vi "set_pixel_dwell_time.vi"(8 "error in (no error)":errorcluster, 10 "Pixel dwell time":dbl=719.0, 11 "TrajectoryRK110428Fiber in":refnum<class "TrajectoryRK110428Fiber_Spiral.lvclass">) -> (0 "error out":errorcluster, 3 "TrajectoryRK110428Fiber out":refnum<class "TrajectoryRK110428Fiber_Spiral.lvclass">)   [LabVIEW 2010, in "TrajectoryRK110428Fiber_Spiral.lvclass"]
uses:
  TrajectoryRK110428Fiber_Spiral.lvclass
  TrajectoryRK110428Fiber_Spiral.lvclass/TrajectoryRK110428Fiber_Spiral.ctl
panel:
  # "[µs]"
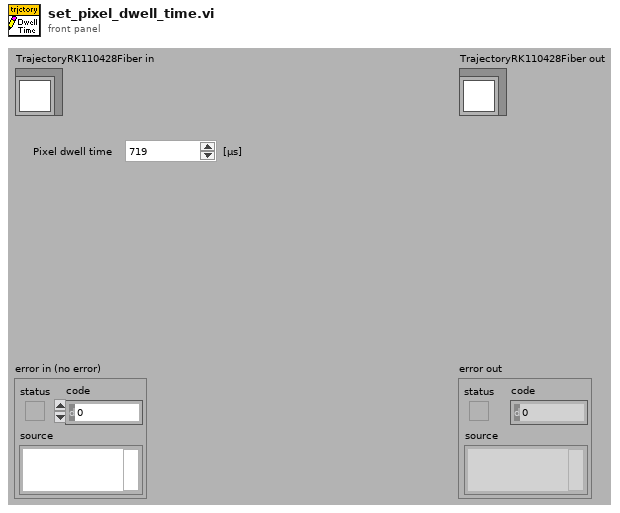
[diagram p1: front panel]
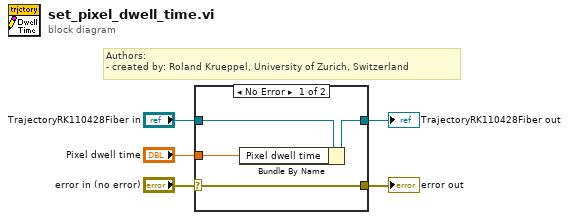
[diagram p0: block diagram]
diagram:
  # "Authors: \n- created by: Roland Krueppel, University of Zurich, Switzerland"
  n1 = case shown="No Error" "error in (no error)" {
    selector: "error in (no error)" -> [w9 w10]
    tunnel: [w9 w10] -> w4
    tunnel: [w7 w11] -> w2
    tunnel: "TrajectoryRK110428Fiber in" -> [w8 w11]
    tunnel: "Pixel dwell time" -> [w6 _]
    frame No Error {
      n2 = Bundle By Name(cluster=w8, "Pixel dwell time"=w6) -> (w7:refnum<class "TrajectoryRK110428Fiber_Spiral.lvclass">)
    }
    frame Error {
    }
  }
  "error out" <- w4
  "TrajectoryRK110428Fiber out" <- w2
